vi "test11-RegisterUnregister_Event.vi"(8 "error in (no error)":errorcluster, 11 "TestCase in":refnum<class "testcase-CSMGlobalLog.lvclass">) -> (0 "error out":errorcluster, 3 "TestCase out":refnum<class "testcase-CSMGlobalLog.lvclass">)   [LabVIEW 2017, in "testcase-CSMGlobalLog.lvclass"]
uses:
  testcase-CSMGlobalLog.lvclass
  testcase-CSMGlobalLog.lvclass/testcase-CSMGlobalLog.ctl
  src/user.lib/_NEVSTOP/Communicable State Machine(CSM)/_Support/Typedef/_CSM_GlobalLog_MSG.ctl
  src/user.lib/_NEVSTOP/Communicable State Machine(CSM)/_Support/Typedef/_CSM_Response Source Message.ctl
  src/user.lib/_NEVSTOP/Communicable State Machine(CSM)/_Support/Typedef/_CSM_GlobalLog_MSG_TYPE.ctl
  c0dc643a-0362-49fc-99f4-5251266ba5a0.vi
  src/user.lib/_NEVSTOP/Communicable State Machine(CSM)/_Support/GlobalEvent/GEvt-Generate with Rule Check.vi
  src/user.lib/_NEVSTOP/Communicable State Machine(CSM)/AdvanceAPI/CSM - Convert Error to Argument.vi
  src/user.lib/_NEVSTOP/Communicable State Machine(CSM)/AdvanceAPI/CSM - Make String Arguments Safe.vi
  src/user.lib/_NEVSTOP/Communicable State Machine(CSM)/AdvanceAPI/CSM - Keywords.vi
  src/user.lib/_NEVSTOP/Communicable State Machine(CSM)/_Support/GlobalEvent/Cache-GEvt Refs.vi
  src/user.lib/_NEVSTOP/Communicable State Machine(CSM)/_Support/GlobalEvent/LogFilter/LogFilter - Check.vi
  src/user.lib/_NEVSTOP/Communicable State Machine(CSM)/_Support/GlobalEvent/LogFilter/LogFilter.lvclass
  <vilib>/addons/_JKI Toolkits/VI Tester/TestCase.llb/TestCase.lvclass
  src/user.lib/_NEVSTOP/Communicable State Machine(CSM)/Communicable State Machine.lvlib
  C:/Program Files (x86)/National Instruments/LabVIEW 2017/vi.lib/addons/_JKI Toolkits/VI Tester/TestCase.llb/TestCase.lvclass
panel:
  out "String cache each loop":string
  out "error out 2":errorcluster
  out "Timed out":bool[](array[boolean])
  out "LoopCount":i32
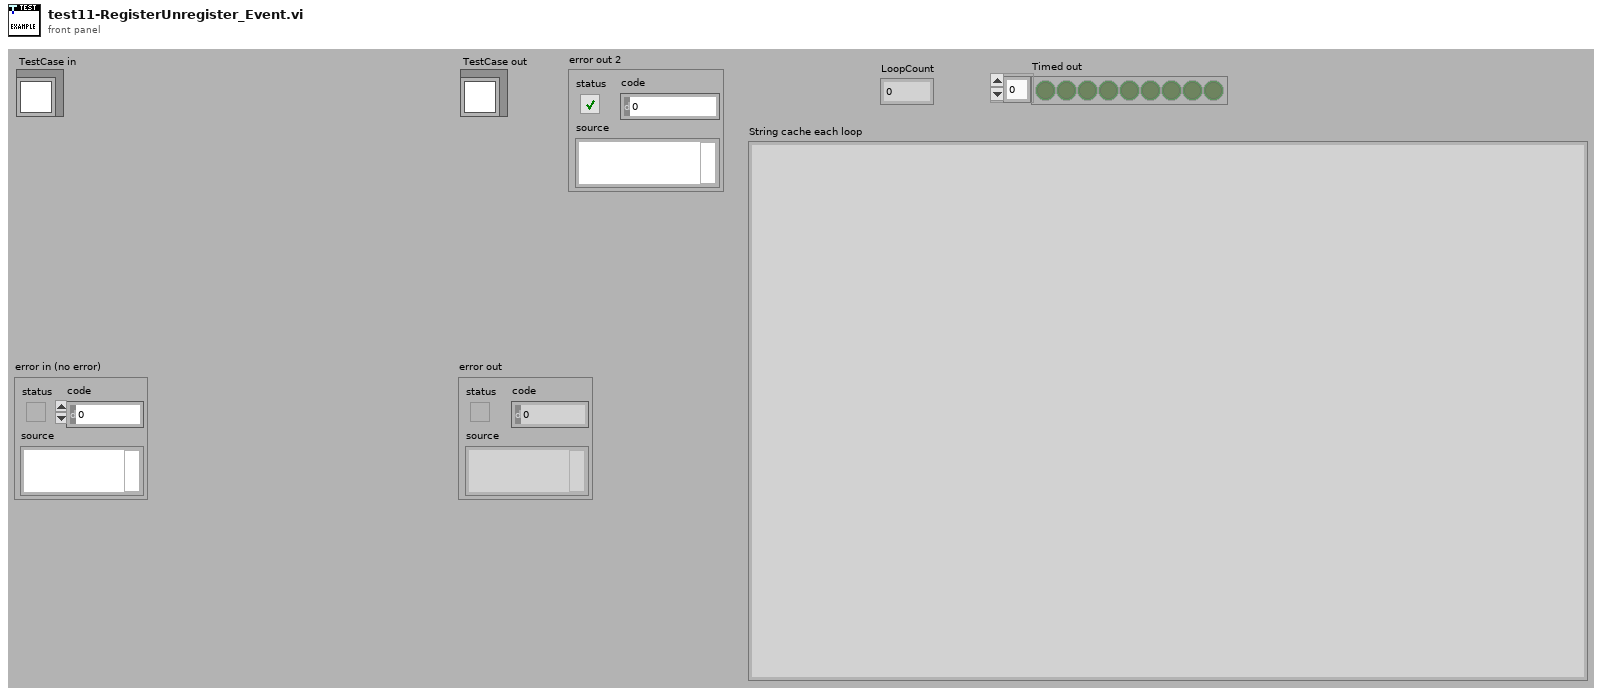
[diagram p1: front panel]
types:
  T1 = typedef "Communicable State Machine.lvlib/_CSM_GlobalLog_MSG.ctl" = cluster{"Name (\"\" to Use UUID)":string, "Current State":string, "Arguments":string, "Source Message":T2, "Source Module":string, "Complete(T)/Start(F)":bool, "LogType":T3, "Time Stamp":timestamp}
  T2 = typedef "Communicable State Machine.lvlib/_CSM_Response Source Message.ctl" = cluster{"‘State":string, "’Arguments":string, "’Error":errorcluster}
  T3 = typedef "Communicable State Machine.lvlib/_CSM_GlobalLog_MSG_TYPE.ctl" = enum16{"User Log", "State Change", "Status", "Interrupt", "Register", "Unregister", "Error Log", "Module Created", "Module Destroyed", "Async Message", "No-Rep Async Message", "Sync Message"}
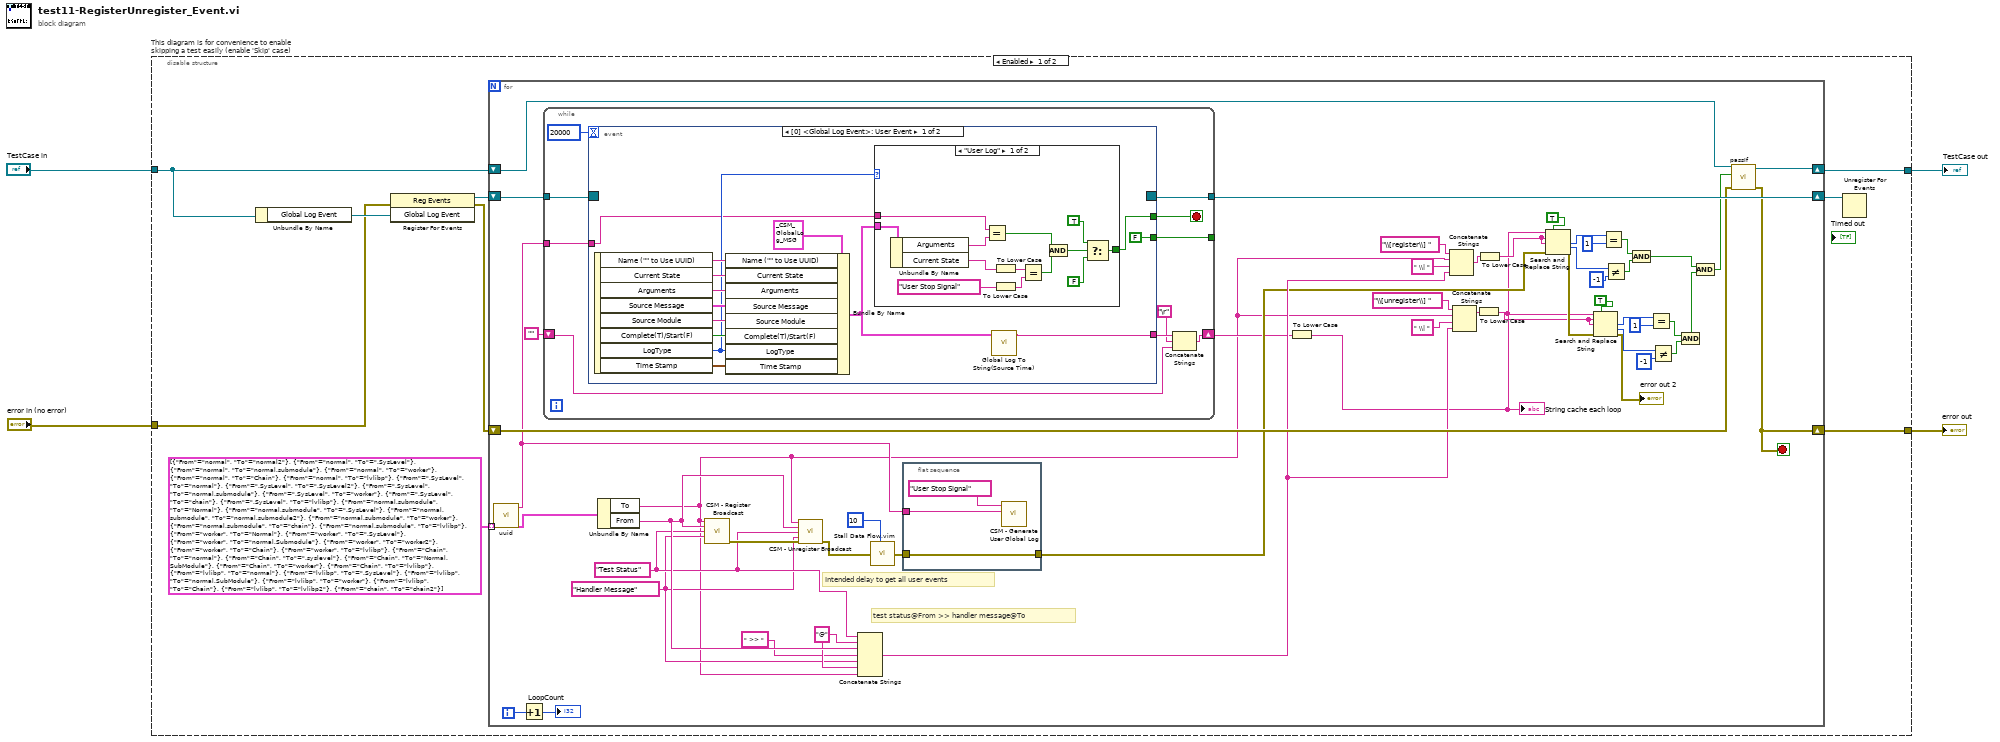
[diagram p0: block diagram]
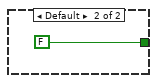
[diagram p2: hidden frame]
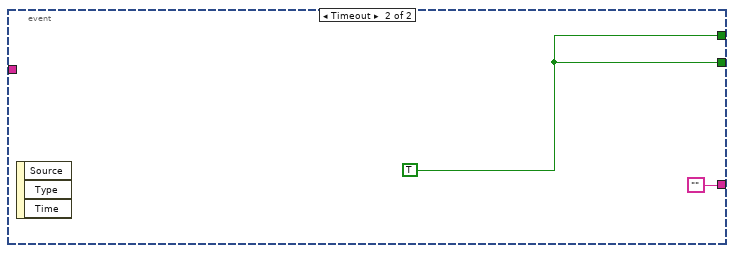
[diagram p3: hidden frame]
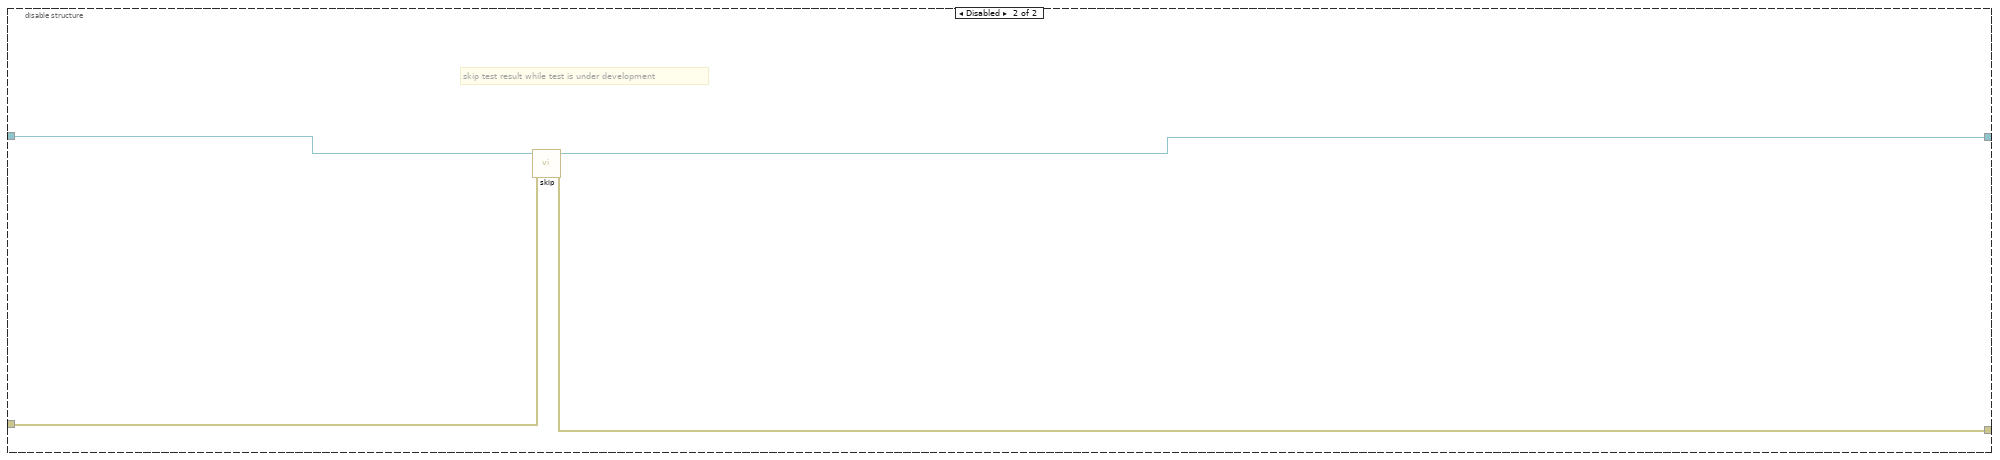
[diagram p4: hidden frame]
diagram:
  n1 = disable-structure "This diagram is for convenience to enable skipping a test easily (enable 'Skip' case)" shown="Enabled" {
    disable-tunnel: "TestCase in" -> [w8 w112]
    disable-tunnel: [w7 w110] -> w1
    disable-tunnel: [w6 w111] -> w3
    disable-tunnel: "error in (no error)" -> [w12 w109]
    frame Enabled {
      n2 = Unbundle By Name(w8) -> ("Global Log Event"=w13:refnum<user-event>)
      n3 = register-events(error in=w12, w13) -> (reference out=w11:refnum<event-registration>, error out=w9:errorcluster)  [unwired: 1 in]
      n4 = for {
        shift-right: [w64] -> w10
        shift-left: w11 -> [w65]
        shift-right: [w60] -> w6
        shift-left: w9 -> [w62]
        tunnel: cluster{"From":string, "To":string}[] [{"From"="normal", "To"="normal2"}, {"From"="normal", "To"=".SysLevel"}, {"From"="normal", "To"="normal.submodule"}, {"From"="normal", "To"="worker"}, {"From"="normal", "To"="Chain"}, {"From"="normal", "To"="lvlibp"}, {"From"=".SysLevel", "To"="normal"}, {"From"=".SysLevel", "To"=".SysLevel2"}, {"From"=".SysLevel", "To"="normal.submodule"}, {"From"=".SysLevel", "To"="worker"}, {"From"=".SysLevel", "To"="chain"}, {"From"=".SysLevel", "To"="lvlibp"}, {"From"="normal.submodule", "To"="Normal"}, {"From"="normal.submodule", "To"=".SysLevel"}, {"From"="normal.submodule", "To"="normal.submodule2"}, {"From"="normal.submodule", "To"="worker"}, {"From"="normal.submodule", "To"="chain"}, {"From"="normal.submodule", "To"="lvlibp"}, {"From"="worker", "To"="Normal"}, {"From"="worker", "To"=".SysLevel"}, {"From"="worker", "To"="normal.Submodule"}, {"From"="worker", "To"="worker2"}, {"From"="worker", "To"="Chain"}, {"From"="worker", "To"="lvlibp"}, {"From"="Chain", "To"="normal"}, {"From"="Chain", "To"=".syslevel"}, {"From"="Chain", "To"="Normal.SubModule"}, {"From"="Chain", "To"="worker"}, {"From"="Chain", "To"="lvlibp"}, {"From"="lvlibp", "To"="normal"}, {"From"="lvlibp", "To"=".SysLevel"}, {"From"="lvlibp", "To"="normal.SubModule"}, {"From"="lvlibp", "To"="worker"}, {"From"="lvlibp", "To"="Chain"}, {"From"="lvlibp", "To"="lvlibp2"}, {"From"="chain", "To"="chain2"}] -> [w23] mode=indexing
        shift-right: [w63] -> w7
        shift-left: w8 -> [w59]
        i -> [w18]
        stop <- w60 stop-if-true
        w36 = "@" ("Trigger")
        w34 = "Handler Message" ("API (If \"\", Same as Trigger)")
        w37 = "Test Status" ("Trigger")
        # "Intended delay to get all user events"
        # "test status@From >> handler message@To"
        n5 = call "uuid.vi"() -> ("UUID"=w20:string)  [unwired: 11 in]
        n6 = Increment(x=w18) -> (x+1=→"LoopCount":i32)
        n7 = while {
          tunnel: w65 -> [w78]
          tunnel: [w77] -> w64
          shift-right: [w69] -> w19
          shift-left: "" -> [w72]
          tunnel: w20 -> [w74]
          tunnel: [w73] -> _
          stop <- w76 stop-if-true
          n8 = event shown="[0] <Global Log Event>: User Event" {
            selector: w78 -> [_ _]
            dyn-events: [_ _] -> w77
            timeout: 20000 -> [_ _]
            tunnel: [w79 ""] -> w71
            tunnel: [w81 w108] -> w76
            tunnel: w74 -> [w82 _]
            tunnel: [FALSE ("Stop") w108] -> w73
            event User Event {
              n9 = event-data() -> ("Name (\"\" to Use UUID)"=w91:string, "Current State"=w90:string, "Arguments"=w89:string, "Source Message"=w88:T2, "Source Module"=w87:string, "Complete(T)/Start(F)"=w86:bool, "LogType"=w83:T3, "Time Stamp"=w85:timestamp)  [unwired: 1 in]
              n10 = Bundle By Name(cluster=T1 {"Name (\"\" to Use UUID)"="", "Current State"="", "Arguments"="", "Source Message"={"‘State"="", "’Arguments"="", "’Error"={"status"=FALSE, "code"=0, "source"=""}}, "Source Module"="", "Complete(T)/Start(F)"=FALSE, "LogType"=enum."State Change", "Time Stamp"=timestamp(0 s since 1904-01-01)} ("Cross CSM Data"), "Name (\"\" to Use UUID)"=w91, "Current State"=w90, "Arguments"=w89, "Source Message"=w88, "Source Module"=w87, "Complete(T)/Start(F)"=w86, "LogType"=w83, "Time Stamp"=w85) -> (w80:T1)
              n11 = case shown="\"User Log\"" w83 {
                tunnel: w80 -> [w105 _]
                tunnel: w82 -> [w104 _]
                tunnel: [w93 FALSE] -> w81
                frame "User Log" {
                  n12 = Unbundle By Name(w105) -> ("Arguments"=w103:string, "Current State"=w102:string)
                  n13 = Equal?(x=w104, y=w103) -> (x = y?=w97:bool)
                  n14 = To Lower Case(string=w102) -> (all lower case string=w101:string)
                  n15 = To Lower Case(string="User Stop Signal" ("Log")) -> (all lower case string=w99:string)
                  n16 = Equal?(x=w101, y=w99) -> (x = y?=w98:bool)
                  n17 = And(x=w97, y=w98) -> (x .and. y?=w96:bool)
                  n18 = Select(t=TRUE, s=w96, f=FALSE) -> (s? t:f=w93:bool)
                }
                frame Default {
                }
              }
              n19 = call "Global Log To String(Source Time).vi"("Log"=w80) -> ("Log String"=w79:string)  [unwired: 9 in]
            }
            event Timeout {
              w108 = TRUE ("Stop")
              n20 = event-data() -> ()  [unwired: 1 in, 3 out]
            }
          }
          n21 = Concatenate Strings(w71, "\r", w72) -> (w69:string)
        }
        n22 = Unbundle By Name(w23) -> ("To"=w16:string, "From"=w55:string)
        n23 = call "CSM - Register Broadcast.vi"("CSM Name(Empty for Broadcast Event)"=w16, "Source CSM Name (* as Default)"=w55, "Trigger"=w37, "API (If \"\", Same as Trigger)"=w34) -> ("error out"=w57:errorcluster)  [unwired: 10 in, 1 out]
        n24 = call "CSM - Unregister Broadcast.vi"("CSM Name(Empty for Broadcast Event)"=w16, "Source CSM Name (* as Default)"=w55, "Trigger"=w37, "API (\"*\" as Default)"=w34, "Error In"=w57) -> ("error out"=w58:errorcluster)  [unwired: 9 in, 1 out]
        n25 = Concatenate Strings(w37, w36, w55, " >> " ("string"), w34, w36, w16) -> (w56:string)
        n26 = call "Stall Data Flow.vim"("value in"=w58, "milliseconds to wait"=u32 10) -> ("value out"=w22:errorcluster)  [unwired: 1 out]
        n27 = flat-sequence {
          tunnel: w20 -> [w67]
          tunnel: w22 -> [w66]
          tunnel: [w66] -> w21
          frame #0 {
            n28 = call "CSM - Generate User Global Log.vi"("Arguments"=w67, "Log"="User Stop Signal") -> ()  [unwired: 9 in, 1 out]
          }
        }
        n29 = To Lower Case(string=w19) -> (all lower case string=w14:string)
        "String cache each loop" <- w14
        n30 = Concatenate Strings("\\[register\\] " ("regular expression"), w16, " \\| " ("string"), w56) -> (w40:string)
        n31 = Concatenate Strings("\\[unregister\\] " ("regular expression"), w16, " \\| " ("string"), w56) -> (w39:string)
        n32 = To Lower Case(string=w39) -> (all lower case string=w50:string)
        n33 = To Lower Case(string=w40) -> (all lower case string=w41:string)
        n34 = Search and Replace String(replace all?=TRUE ("replace all? (F)"), input string=w14, search string=w41, replace string=w41, error in=w21) -> (number of replacements=w42:i32, offset past replacement=w43:i32, error out=w51:errorcluster)  [unwired: 3 in, 1 out]
        n35 = Search and Replace String(replace all?=TRUE ("replace all? (F)"), input string=w14, search string=w50, replace string=w50, error in=w51) -> (number of replacements=w49:i32, offset past replacement=w48:i32, error out=→"error out 2":errorcluster)  [unwired: 3 in, 1 out]
        n36 = Equal?(x=w42, y=1) -> (x = y?=w44:bool)
        n37 = Not Equal?(x=w43, y=-1) -> (x != y?=w45:bool)
        n38 = And(x=w44, y=w45) -> (x .and. y?=w54:bool)
        n39 = Equal?(x=w49, y=1) -> (x = y?=w47:bool)
        n40 = Not Equal?(x=w48, y=-1) -> (x != y?=w46:bool)
        n41 = And(x=w47, y=w46) -> (x .and. y?=w52:bool)
        n42 = And(x=w54, y=w52) -> (x .and. y?=w17:bool)
        n43 = call-dynamic "passIf.vi"("error in (no error)"=w62, "pass"=w17, "TestCase in"=w59) -> ("error out"=w60:errorcluster, "TestCase out"=w63:refnum<class "testcase-CSMGlobalLog.lvclass">)  [unwired: 7 in]
      }
      n44 = Unregister For Events(event registration refnum=w10) -> ()  [unwired: 1 in, 1 out]
    }
    frame Disabled {
      # "skip test result while test is under development"
      n45 = call <vilib>:"skip.vi"("error in (no error)"=w109, "TestCase in"=w112) -> ("error out"=w111:errorcluster, "TestCase out"=w110:refnum<class "testcase-CSMGlobalLog.lvclass">)  [unwired: 8 in]
    }
  }
  "error out" <- w3
  "TestCase out" <- w1
